vi "SDSU_GetClkType.vi"(10 "TableIn":string[][](table), 11 "type":string) -> (2 "Table Out":string[][](table))   [LabVIEW 2016]
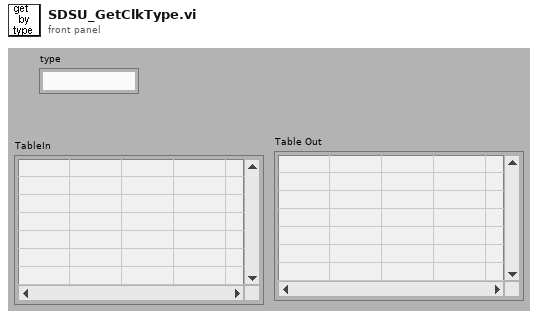
[diagram p1: front panel]
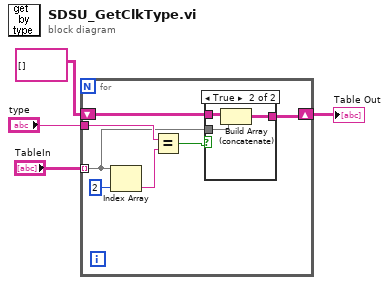
[diagram p0: block diagram]
diagram:
  n1 = for {
    tunnel: "TableIn" -> [w7] mode=indexing
    tunnel: "type" -> [w10]
    shift-right: [w6] -> w2
    shift-left: string[][] [] -> [w5]
    n2 = Index Array(array=w7, index=2) -> (element=w9:string)
    n3 = Equal?(x=w10, y=w9) -> (x = y?=w8:bool)
    n4 = case shown="True" w8 {
      tunnel: w7 -> [_ w15]
      tunnel: [w12 w14] -> w6
      tunnel: w5 -> [w12 w13]
      frame False {
      }
      frame True {
        n5 = Build Array (concatenate)(w13, w15) -> (w14:string[][])
      }
    }
  }
  "Table Out" <- w2
